vi "ConfigureCurrentController.vi"(0 "axis in":cluster{"keyHandle":u32, "nodeId":u16}={"keyHandle"=0, "nodeId"=1}, 9 "current gains":cluster{"p-Gain":u64, "i-Gain":u64}, 11 "error in (no error)":errorcluster) -> (4 "axis out":cluster{"keyHandle":u32, "nodeId":u16}={"keyHandle"=0, "nodeId"=1}, 15 "error out":errorcluster)   [LabVIEW 2019, in "maxonEPOS.lvlib"]
doc: "<B>ConfigureCurrentRegulator</B> writes the current regulation gain parameters to the device."
uses:
  Examples/maxonEPOS.lvlib
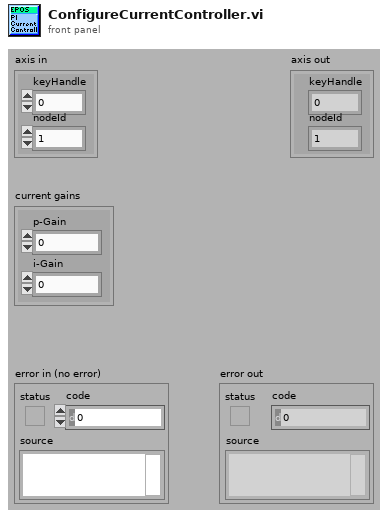
[diagram p1: front panel]
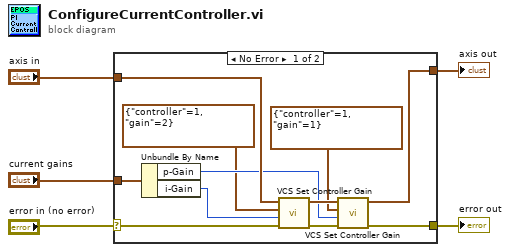
[diagram p0: block diagram]
diagram:
  n1 = case shown="No Error" "error in (no error)" {
    selector: "error in (no error)" -> [w15 w18]
    tunnel: [w13 w18] -> w4
    tunnel: [w14 w17] -> w3
    tunnel: "axis in" -> [w16 w17]
    tunnel: "current gains" -> [w10 _]
    frame No Error {
      n2 = Unbundle By Name(w10) -> ("p-Gain"=w8:u64, "i-Gain"=w9:u64)
      n3 = call "VCS Set Controller Gain.vi"("error in (no error)"=w15, "value"=w9, "controller gain"=cluster{"controller":u16, "gain":u16} {"controller"=1, "gain"=2}, "axis in"=w16) -> ("error out"=w12:errorcluster, "axis out"=w11:cluster{"keyHandle":u32, "nodeId":u16})  [unwired: 6 in]
      n4 = call "VCS Set Controller Gain.vi"("error in (no error)"=w12, "value"=w8, "controller gain"=cluster{"controller":u16, "gain":u16} {"controller"=1, "gain"=1}, "axis in"=w11) -> ("error out"=w13:errorcluster, "axis out"=w14:cluster{"keyHandle":u32, "nodeId":u16})  [unwired: 6 in]
    }
    frame Error {
    }
  }
  "error out" <- w4
  "axis out" <- w3
